vi "Terminal Menu Actor - Account Action Completed.vi"   [LabVIEW 2016, in "CLD Exam - ATM.lvlib"]
uses:
  CLD Exam - ATM.lvlib
  Mediator/Classes/Message Transport Event/Message Transport Event.lvclass
  D:/Repos/Stream/software/Mediator/Classes/Message Transport Interface/Message Transport Interface.lvclass
  Mediator/Classes/Message Broker Interface Ref/Message Broker Interface Ref.lvclass
  Classes/Terminal Menus/Terminal Menus.lvclass
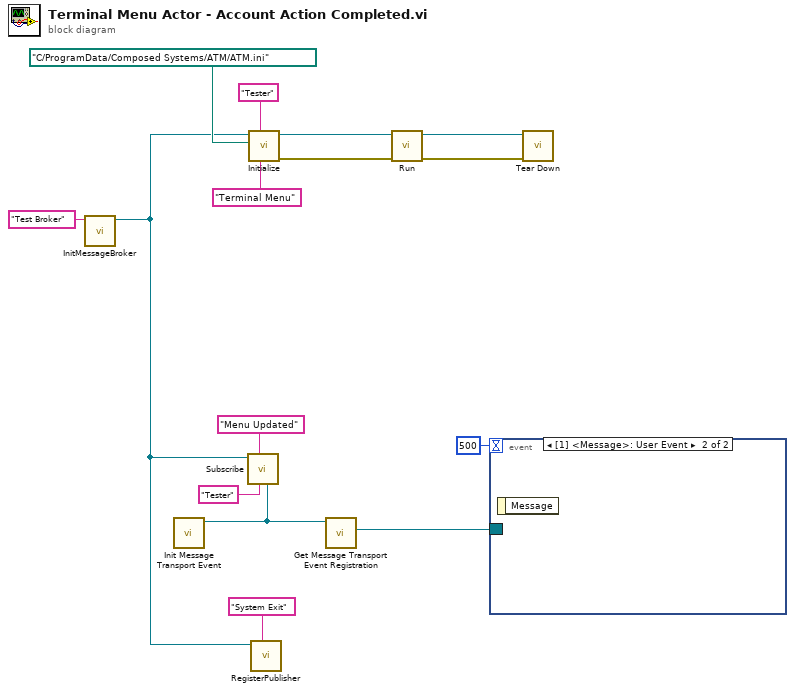
[diagram p0: block diagram]
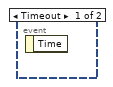
[diagram p2: hidden frame]
diagram:
  n1 = call "InitMessageBroker.vi"("Broker Name"="Test Broker") -> ("Message Broker Interface Ref out"=w5:refnum<class "Message Broker Interface Ref.lvclass">)  [unwired: 9 in, 1 out]
  n2 = call "Init Message Transport Event.vi"() -> ("Message Transport Event out"=w8:refnum<class "Message Transport Event.lvclass">)  [unwired: 10 in, 1 out]
  n3 = call-dynamic "Subscribe.vi"("Message Transport Interface"=w8, "Subscriber Name"="Tester", "Topic Name"="Menu Updated", "Message Broker Interface TAP in"=w5) -> ()  [unwired: 5 in, 3 out]
  n4 = call "Initialize.vi"("Actor Name"="Terminal Menu", "Host Name"="Tester", "Application Data"=path "C:/ProgramData/Composed Systems/ATM/ATM.ini", "Message Broker"=w5) -> ("error out"=w10:errorcluster, "Terminal Menus out"=w11:refnum<class "Terminal Menus.lvclass">)  [unwired: 6 in]
  n5 = call-dynamic "RegisterPublisher.vi"("Topic Name"="System Exit", "Message Broker Interface Ref in"=w5) -> ()  [unwired: 5 in, 5 out]
  n6 = call "Get Message Transport Event Registration.vi"("Message Transport Event in"=w8) -> ("Event Registration Refnum"=w4:refnum<event-registration>)  [unwired: 7 in, 3 out]
  n7 = call-dynamic "Run.vi"("error in (no error)"=w10, "Terminal Menus in"=w11) -> ("error out"=w1:errorcluster, "Terminal Menus out"=w2:refnum<class "Terminal Menus.lvclass">)  [unwired: 8 in]
  n8 = event shown="[1] <Message>: User Event" {
    selector: w4 -> [_ _]
    dyn-events: _ -> [_ _]
    timeout: 500 -> [_ _]
    event Timeout {
      n9 = event-data() -> ()  [unwired: 1 in, 1 out]
    }
    event User Event {
      n10 = event-data() -> ()  [unwired: 1 in, 1 out]
    }
  }
  n11 = call "Tear Down.vi"("error in (no error)"=w1, "Terminal Menus in"=w2) -> ()  [unwired: 8 in, 2 out]
